vi "Pull GUI References.vi"(8 "error in":errorcluster, 11 "Base Software in":refnum<class "Main.lvclass">) -> (0 "error out":errorcluster, 3 "Base Software out":refnum<class "Main.lvclass">)   [LabVIEW 2023, in "Main.lvlib" / "Main.lvclass"]
uses:
  Project/Main.lvclass
  C:/Users/Public/Documents/Development/builds/Engine/Engine.lvlibp/Project/Engine.lvclass
  Project/Main.lvclass/Main.ctl
  Accessors/StateMachine/Write UUT_Info.vi
  builds/Engine/Engine.lvlibp/Methods/Read Revision.vi
  builds/Engine/Engine.lvlibp/Accessors/Read VI_Ref.vi
  Events/Log On.vi
  Accessors/Indicators/Write Model.vi
  Accessors/Indicators/Write Serial.vi
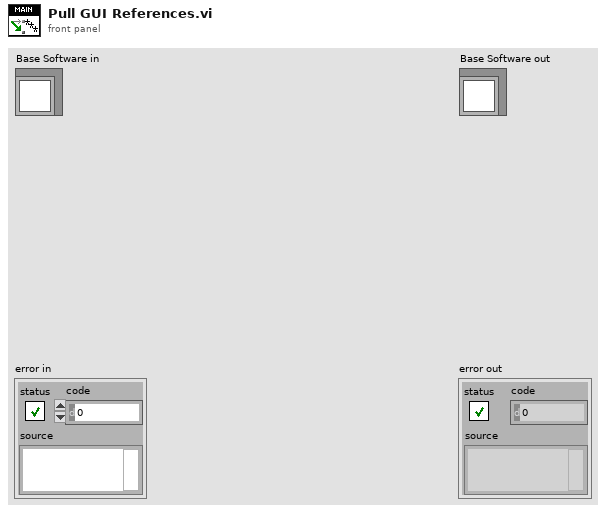
[diagram p1: front panel]
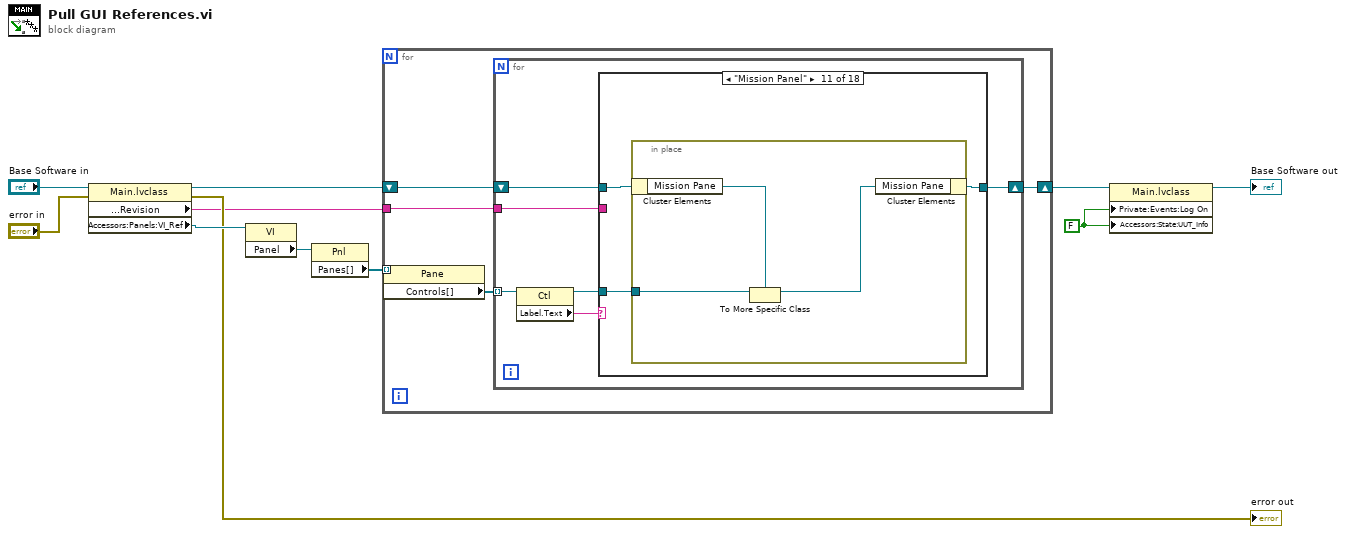
[diagram p0: block diagram]
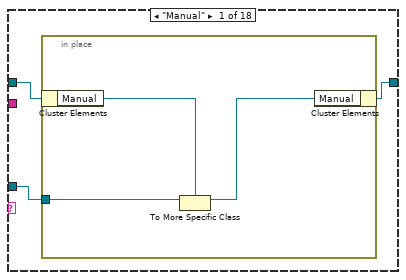
[diagram p2: hidden frame]
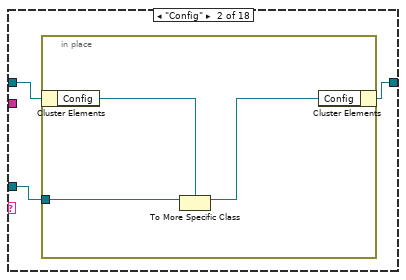
[diagram p3: hidden frame]
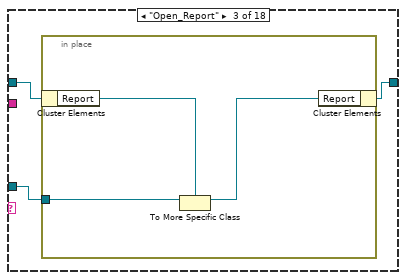
[diagram p4: hidden frame]
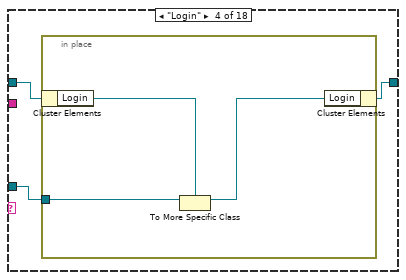
[diagram p5: hidden frame]
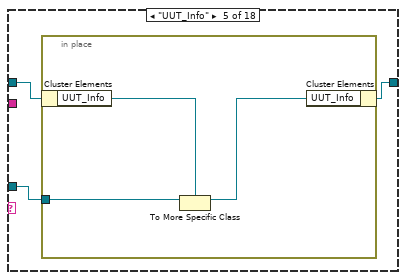
[diagram p6: hidden frame]
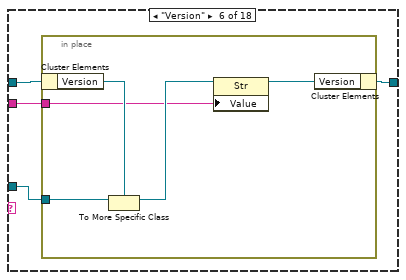
[diagram p7: hidden frame]
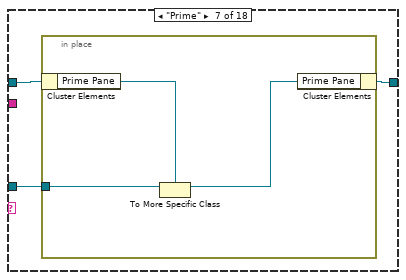
[diagram p8: hidden frame]
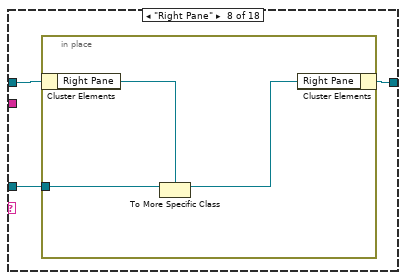
[diagram p9: hidden frame]
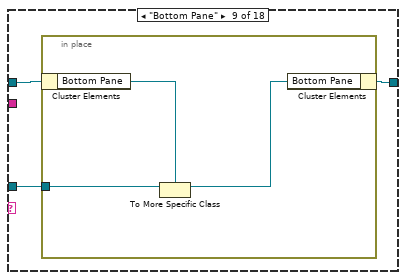
[diagram p10: hidden frame]
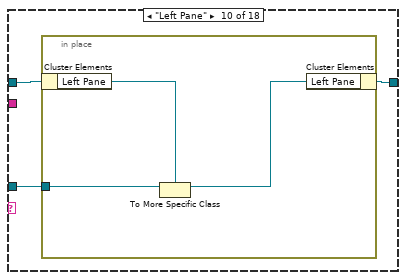
[diagram p11: hidden frame]
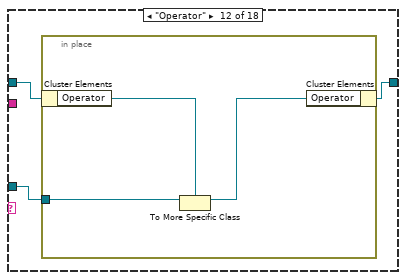
[diagram p12: hidden frame]
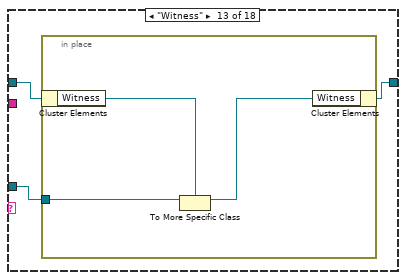
[diagram p13: hidden frame]
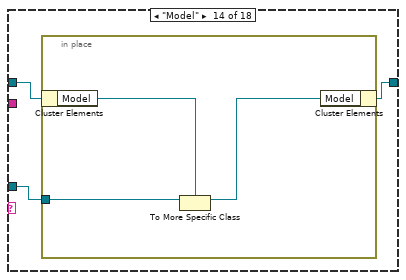
[diagram p14: hidden frame]
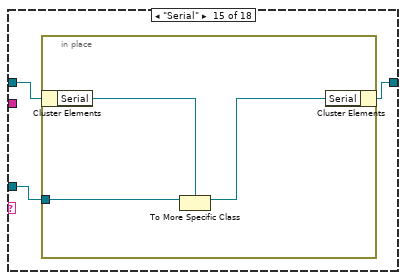
[diagram p15: hidden frame]
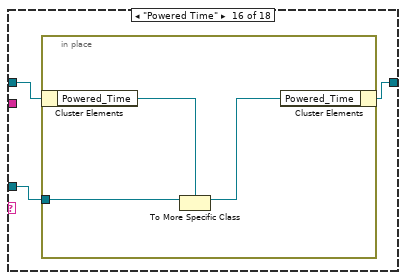
[diagram p16: hidden frame]
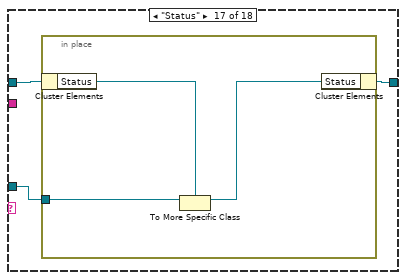
[diagram p17: hidden frame]
diagram:
  w1 = FALSE ("Base:StateMachine:UUT_Info")
  n1 = property class="Main.lvclass"(reference="Base Software in", error in="error in") -> (reference out=w8:refnum<class "Main.lvclass">, error out=→"error out":errorcluster, "Accessors:Application:Information:Revision"=w6:string, "Accessors:Panels:VI_Ref"=w10:refnum<vi>)
  n2 = property class="VI"(reference=w10) -> ("Panel"=w9:refnum<vi>)  [unwired: 1 in, 2 out]
  n3 = property class="Pnl"(reference=w9) -> ("Panes[]"=w4:refnum<vi>[])  [unwired: 1 in, 2 out]
  n4 = for {
    shift-right: [w15] -> w3
    shift-left: w8 -> [w16]
    tunnel: w6 -> [w14]
    tunnel: w4 -> [w12] mode=indexing
    n5 = property class="Pane"(reference=w12) -> ("Controls[]"=w13:refnum<vi>[])  [unwired: 1 in, 2 out]
    n6 = for {
      tunnel: w13 -> [w22] mode=indexing
      tunnel: w14 -> [w17]
      shift-right: [w19] -> w15
      shift-left: w16 -> [w20]
      n7 = property class="Ctl"(reference=w22) -> (reference out=w18:refnum<vi>, "Label.Text"=w21:string)  [unwired: 1 in, 1 out]
      n8 = case shown="\"Mission Panel\"" w21 {
        tunnel: w20 -> [w25 w31 w37 w43 w49 w56 w64 w70 w76 w82 w88 w94 w100 w106 w112 w118 w124 w128]
        tunnel: [w24 w30 w36 w42 w48 w55 w63 w69 w75 w81 w87 w93 w99 w105 w111 w117 w123 w128] -> w19
        tunnel: w18 -> [w23 w29 w35 w41 w47 w54 w62 w68 w74 w80 w86 w92 w98 w104 w110 w116 w122 _]
        tunnel: w17 -> [_ _ _ _ _ w53 _ _ _ _ _ _ _ _ _ _ _ _]
        frame "Manual" {
          n9 = in-place {
            in-place-border: w23 -> [w28]
            n10 = in-place-cluster #1(w25) -> ("Manual"=w27:refnum<vi>)
            n11 = To More Specific Class(target class=w27, reference=w28) -> (specific class reference=w26:refnum<vi>)  [unwired: 1 in, 1 out]
            n12 = in-place-cluster #1("Manual"=w26) -> (w24:refnum<class "Main.lvclass">)
          }
        }
        frame "Config" {
          n13 = in-place {
            in-place-border: w29 -> [w34]
            n14 = in-place-cluster #2(w31) -> ("Config"=w33:refnum<vi>)
            n15 = To More Specific Class(target class=w33, reference=w34) -> (specific class reference=w32:refnum<vi>)  [unwired: 1 in, 1 out]
            n16 = in-place-cluster #2("Config"=w32) -> (w30:refnum<class "Main.lvclass">)
          }
        }
        frame "Open_Report" {
          n17 = in-place {
            in-place-border: w35 -> [w40]
            n18 = in-place-cluster #3(w37) -> ("Report"=w39:refnum<vi>)
            n19 = To More Specific Class(target class=w39, reference=w40) -> (specific class reference=w38:refnum<vi>)  [unwired: 1 in, 1 out]
            n20 = in-place-cluster #3("Report"=w38) -> (w36:refnum<class "Main.lvclass">)
          }
        }
        frame "Login" {
          n21 = in-place {
            in-place-border: w41 -> [w46]
            n22 = in-place-cluster #4(w43) -> ("Login"=w45:refnum<vi>)
            n23 = To More Specific Class(target class=w45, reference=w46) -> (specific class reference=w44:refnum<vi>)  [unwired: 1 in, 1 out]
            n24 = in-place-cluster #4("Login"=w44) -> (w42:refnum<class "Main.lvclass">)
          }
        }
        frame "UUT_Info" {
          n25 = in-place {
            in-place-border: w47 -> [w52]
            n26 = in-place-cluster #5(w49) -> ("UUT_Info"=w51:refnum<vi>)
            n27 = To More Specific Class(target class=w51, reference=w52) -> (specific class reference=w50:refnum<vi>)  [unwired: 1 in, 1 out]
            n28 = in-place-cluster #5("UUT_Info"=w50) -> (w48:refnum<class "Main.lvclass">)
          }
        }
        frame "Version" {
          n29 = in-place {
            in-place-border: w54 -> [w61]
            in-place-border: w53 -> [w57]
            n30 = in-place-cluster #6(w56) -> ("Version"=w60:refnum<vi>)
            n31 = To More Specific Class(target class=w60, reference=w61) -> (specific class reference=w59:refnum<vi>)  [unwired: 1 in, 1 out]
            n32 = property class="Str"(reference=w59, "Value"=w57) -> (reference out=w58:refnum<vi>)  [unwired: 1 in, 1 out]
            n33 = in-place-cluster #6("Version"=w58) -> (w55:refnum<class "Main.lvclass">)
          }
        }
        frame "Prime" {
          n34 = in-place {
            in-place-border: w62 -> [w67]
            n35 = in-place-cluster #7(w64) -> ("Prime Pane"=w66:refnum<vi>)
            n36 = To More Specific Class(target class=w66, reference=w67) -> (specific class reference=w65:refnum<vi>)  [unwired: 1 in, 1 out]
            n37 = in-place-cluster #7("Prime Pane"=w65) -> (w63:refnum<class "Main.lvclass">)
          }
        }
        frame "Right Pane" {
          n38 = in-place {
            in-place-border: w68 -> [w73]
            n39 = in-place-cluster #8(w70) -> ("Right Pane"=w72:refnum<vi>)
            n40 = To More Specific Class(target class=w72, reference=w73) -> (specific class reference=w71:refnum<vi>)  [unwired: 1 in, 1 out]
            n41 = in-place-cluster #8("Right Pane"=w71) -> (w69:refnum<class "Main.lvclass">)
          }
        }
        frame "Bottom Pane" {
          n42 = in-place {
            in-place-border: w74 -> [w79]
            n43 = in-place-cluster #9(w76) -> ("Bottom Pane"=w78:refnum<vi>)
            n44 = To More Specific Class(target class=w78, reference=w79) -> (specific class reference=w77:refnum<vi>)  [unwired: 1 in, 1 out]
            n45 = in-place-cluster #9("Bottom Pane"=w77) -> (w75:refnum<class "Main.lvclass">)
          }
        }
        frame "Left Pane" {
          n46 = in-place {
            in-place-border: w80 -> [w85]
            n47 = in-place-cluster #10(w82) -> ("Left Pane"=w84:refnum<vi>)
            n48 = To More Specific Class(target class=w84, reference=w85) -> (specific class reference=w83:refnum<vi>)  [unwired: 1 in, 1 out]
            n49 = in-place-cluster #10("Left Pane"=w83) -> (w81:refnum<class "Main.lvclass">)
          }
        }
        frame "Mission Panel" {
          n50 = in-place {
            in-place-border: w86 -> [w91]
            n51 = in-place-cluster #11(w88) -> ("Mission Pane"=w90:refnum<vi>)
            n52 = To More Specific Class(target class=w90, reference=w91) -> (specific class reference=w89:refnum<vi>)  [unwired: 1 in, 1 out]
            n53 = in-place-cluster #11("Mission Pane"=w89) -> (w87:refnum<class "Main.lvclass">)
          }
        }
        frame "Operator" {
          n54 = in-place {
            in-place-border: w92 -> [w97]
            n55 = in-place-cluster #12(w94) -> ("Operator"=w96:refnum<vi>)
            n56 = To More Specific Class(target class=w96, reference=w97) -> (specific class reference=w95:refnum<vi>)  [unwired: 1 in, 1 out]
            n57 = in-place-cluster #12("Operator"=w95) -> (w93:refnum<class "Main.lvclass">)
          }
        }
        frame "Witness" {
          n58 = in-place {
            in-place-border: w98 -> [w103]
            n59 = in-place-cluster #13(w100) -> ("Witness"=w102:refnum<vi>)
            n60 = To More Specific Class(target class=w102, reference=w103) -> (specific class reference=w101:refnum<vi>)  [unwired: 1 in, 1 out]
            n61 = in-place-cluster #13("Witness"=w101) -> (w99:refnum<class "Main.lvclass">)
          }
        }
        frame "Model" {
          n62 = in-place {
            in-place-border: w104 -> [w109]
            n63 = in-place-cluster #14(w106) -> ("Model"=w108:refnum<vi>)
            n64 = To More Specific Class(target class=w108, reference=w109) -> (specific class reference=w107:refnum<vi>)  [unwired: 1 in, 1 out]
            n65 = in-place-cluster #14("Model"=w107) -> (w105:refnum<class "Main.lvclass">)
          }
        }
        frame "Serial" {
          n66 = in-place {
            in-place-border: w110 -> [w115]
            n67 = in-place-cluster #15(w112) -> ("Serial"=w114:refnum<vi>)
            n68 = To More Specific Class(target class=w114, reference=w115) -> (specific class reference=w113:refnum<vi>)  [unwired: 1 in, 1 out]
            n69 = in-place-cluster #15("Serial"=w113) -> (w111:refnum<class "Main.lvclass">)
          }
        }
        frame "Powered Time" {
          n70 = in-place {
            in-place-border: w116 -> [w121]
            n71 = in-place-cluster #16(w118) -> ("Powered_Time"=w120:refnum<vi>)
            n72 = To More Specific Class(target class=w120, reference=w121) -> (specific class reference=w119:refnum<vi>)  [unwired: 1 in, 1 out]
            n73 = in-place-cluster #16("Powered_Time"=w119) -> (w117:refnum<class "Main.lvclass">)
          }
        }
        frame "Status" {
          n74 = in-place {
            in-place-border: w122 -> [w127]
            n75 = in-place-cluster #17(w124) -> ("Status"=w126:refnum<vi>)
            n76 = To More Specific Class(target class=w126, reference=w127) -> (specific class reference=w125:refnum<vi>)  [unwired: 1 in, 1 out]
            n77 = in-place-cluster #17("Status"=w125) -> (w123:refnum<class "Main.lvclass">)
          }
        }
        frame Default {
        }
      }
    }
  }
  n78 = property class="Main.lvclass"(reference=w3, "Private:Events:Log On"=w1, "Accessors:State:UUT_Info"=w1) -> (reference out=→"Base Software out":refnum<class "Main.lvclass">)  [unwired: 1 in, 1 out]
